vi "Exp6-Simulation.vi"() -> ()   [LabVIEW 2022 SP3]
uses:
  <vilib>/addons/Modulation/Analog/support/mod_Set Error Source.vi
  <vilib>/addons/Modulation/Digital/Support/Common/Validators/mod_AWGN Validate.vi
  <vilib>/addons/Modulation/Digital/Impairments/subVIs/mod_createSeeds.vi
  <vilib>/addons/Modulation/Digital/Support/Common/Validators/mod_Validate Samples Per Symbol.vi
  <vilib>/addons/Modulation/Analog/support/Validators/mod_Validate Complex Waveform.vi
  <vilib>/addons/Modulation/Analog/support/Validators/mod_WFErrorHandler.vi
  <vilib>/addons/Modulation/Digital/General/subVIs/mod_Generate Bits PN Sequence.vi
  <vilib>/Analysis/1siggen.llb/Gaussian White Noise (obs 90).vi
  <vilib>/addons/Modulation/Digital/Support/Common/Validators/mod_Generate Filter Coefficients Validate.vi
  <vilib>/addons/Modulation/Digital/General/subVIs/mod_Generate Filter Coefficients.vi
  <vilib>/addons/Modulation/Digital/General/MT Format Eye Diagram (complex).vi
  <vilib>/addons/Modulation/niDMT.lvlib
panel:
  out "Waveform Graph":cluster{"t0":dbl, "dt":dbl, "Y":dbl[]}[](graph)
  in  "filter parameter":dbl=0.5 format="%.2f"
  in  "M-QAM Demodulate":i32=16
  out "XY Graph 2":T1(graph)
  out "modulated bitstream":i8[](array[numeric])
  out "Waveform":cluster{"t0":dbl, "dt":dbl, "Y":dbl[]}(graph)
  out "Real":cluster{"t0":dbl, "dt":dbl, "Y":dbl[]}(graph)
  out "Imaginary":cluster{"t0":dbl, "dt":dbl, "Y":dbl[]}(graph)
  out "XY Graph":T1(graph)
  in  "M-QAM Modulate":i32=16
  in  "PN Sequence Order":i32=9
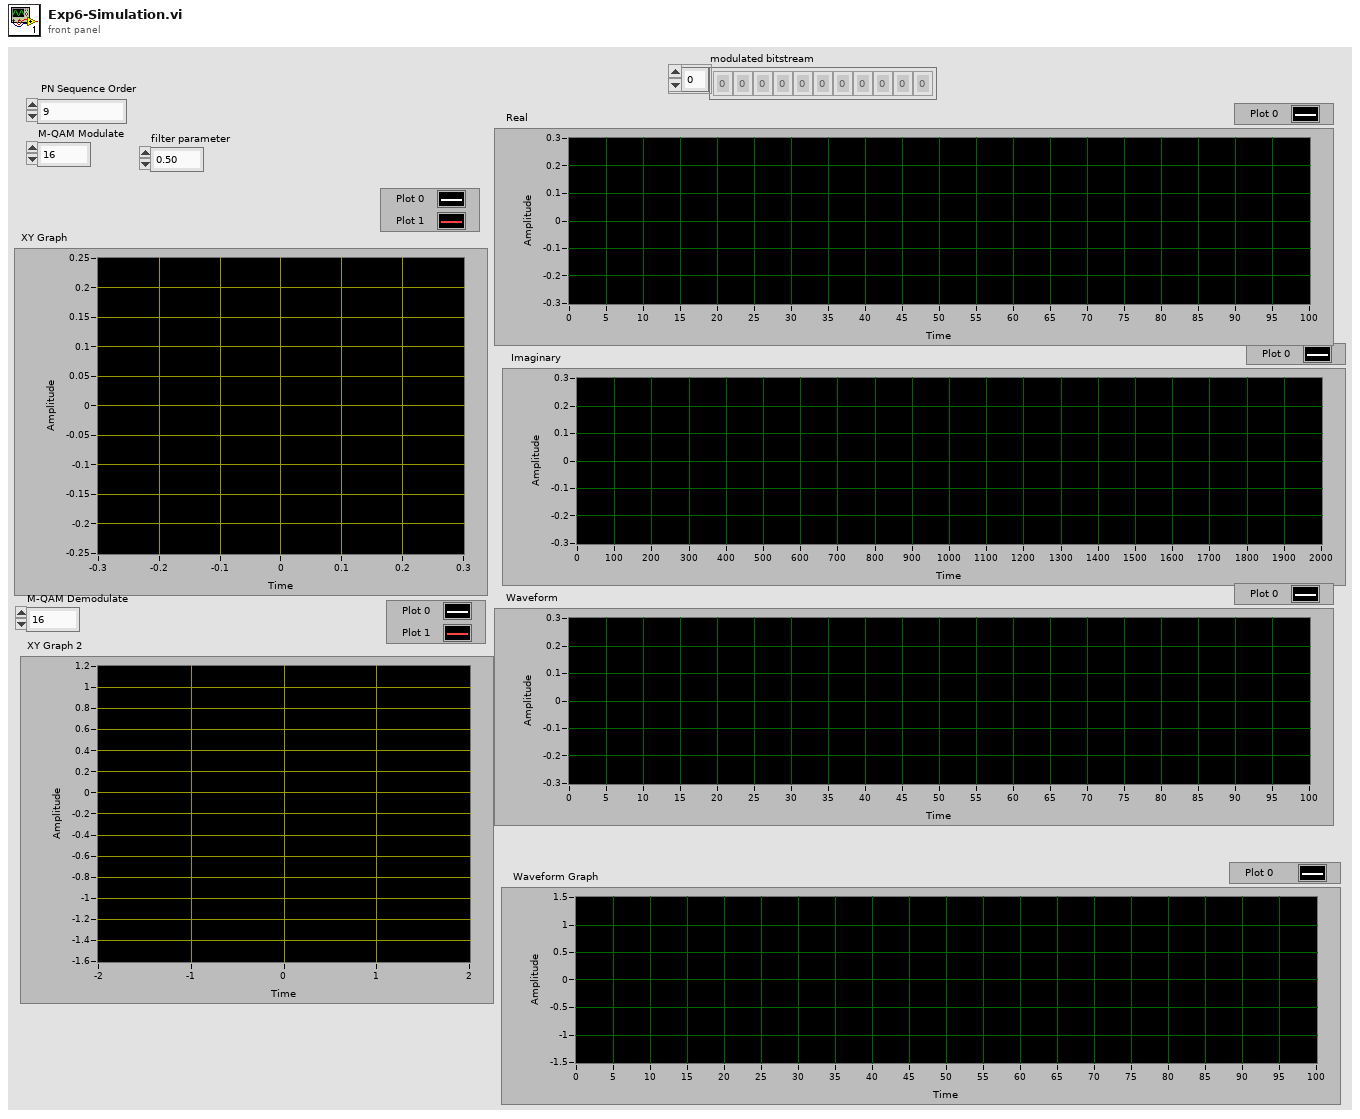
[diagram p1: front panel]
types:
  T1 = cluster{"constellation":dbl[], "oversampled data":dbl[]}[]
  T2 = enum16{"FSK", "PSK", "QAM", "MSK", "PAM", "ASK", "CPM"}
  T3 = enum16{"none", "Raised Cosine", "Root Raised Cos", "Gaussian"}
  T4 = enum32{"PN sequence", "User-defined pattern", "Read from file"}
  T5 = cluster{"samples per symbol (16)":i32, "symbol map":cdb[]}
  T6 = typedef "niAMT.lvlib/Complex Data Waveform.ctl" = cluster{"t0":dbl, "dt":dbl, "Y":cdb[]}
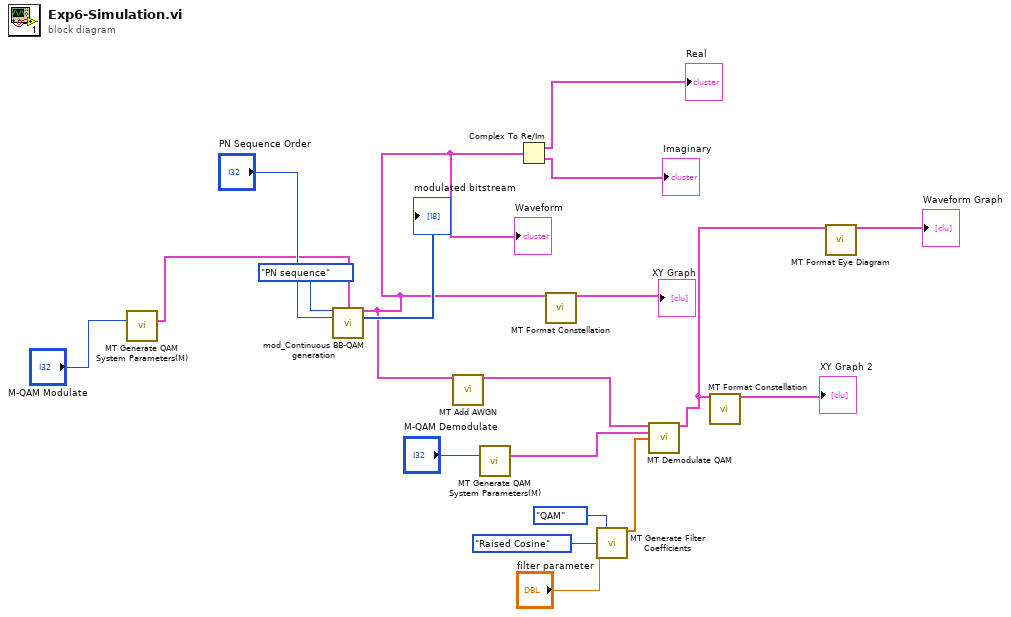
[diagram p0: block diagram]
diagram:
  n1 = call <vilib>:"MT Generate QAM System Parameters(M).vi"("M-QAM (16)"="M-QAM Modulate") -> ("QAM system parameters"=w17:T5)  [unwired: 12 in, 2 out]
  n2 = call <vilib>:"mod_Continuous BB-QAM generation.vi"("Bit stream"=T4."PN sequence", "QAM system parameters"=w17, "PN Sequence Order"="PN Sequence Order") -> ("output complex waveform"=w11:T6, "modulated bitstream"=→"modulated bitstream":i8[])  [unwired: 8 in, 3 out]
  "Waveform" <- w11
  n3 = call <vilib>:"MT Add AWGN.vi"("input complex waveform"=w11) -> ("output complex waveform"=w10:T6)  [unwired: 12 in, 2 out]
  n4 = call <vilib>:"MT Generate QAM System Parameters(M).vi"("M-QAM (16)"="M-QAM Demodulate") -> ("QAM system parameters"=w9:T5)  [unwired: 12 in, 2 out]
  n5 = Complex To Re/Im(x + iy=w11) -> (x=→"Real":cluster{"t0":dbl, "dt":dbl, "Y":dbl[]}, y=→"Imaginary":cluster{"t0":dbl, "dt":dbl, "Y":dbl[]})
  n6 = call <vilib>:"MT Format Constellation.vi"("waveform"=w11) -> ("constellation graph"=→"XY Graph":T1)  [unwired: 13 in, 1 out]
  n7 = call <vilib>:"MT Generate Filter Coefficients.vi"("pulse shaping filter (none)"=T3."Raised Cosine", "modulation type"=T2."QAM", "filter parameter"="filter parameter") -> ("pulse shaping filter coefficients"=w4:dbl[])  [unwired: 10 in, 2 out]
  n8 = call <vilib>:"MT Demodulate QAM.vi"("input complex waveform"=w10, "QAM system parameters"=w9, "matched filter coefficients"=w4) -> ("recovered complex waveform"=w2:T6)  [unwired: 8 in, 4 out]
  n9 = call <vilib>:"MT Format Constellation.vi"("waveform"=w2) -> ("constellation graph"=→"XY Graph 2":T1)  [unwired: 13 in, 1 out]
  n10 = call-poly <vilib>:"MT Format Eye Diagram.vi"("waveform"=w2) -> ("eye diagram"=→"Waveform Graph":cluster{"t0":dbl, "dt":dbl, "Y":dbl[]}[])  [unwired: 13 in, 1 out]
